vi "Stop.vi"(8 "error in (no error)":errorcluster, 11 "MicronManager in":refnum<class "MicronManager.lvclass">) -> (0 "error out":errorcluster, 3 "MicronManager out":refnum<class "MicronManager.lvclass">)   [LabVIEW 2019, in "MicronManager.lvclass"]
uses:
  MicronManager.lvclass
  MicronManager.lvclass/MicronManager.ctl
  <vilib>/SLL Toolkit/SLL Easy TCP/_SubVIs/TCP Initialize Client - Local.vi
  <vilib>/SLL Toolkit/SLL Easy TCP/SLL Easy API via TCP.lvclass
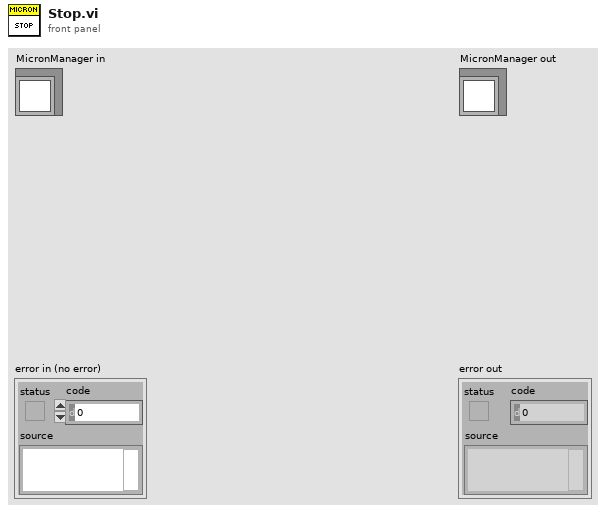
[diagram p1: front panel]
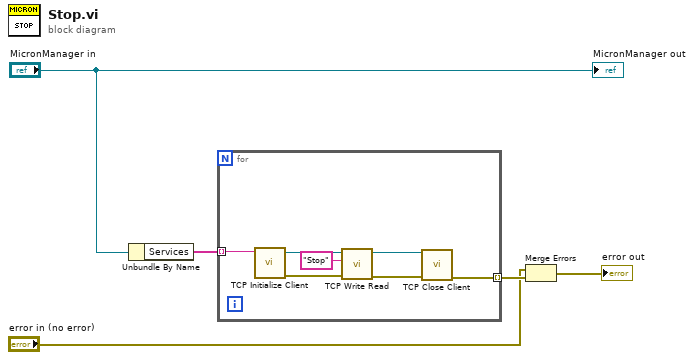
[diagram p0: block diagram]
diagram:
  n1 = Unbundle By Name("MicronManager in") -> ("Services"=w1:string[])
  n2 = for {
    tunnel: w1 -> [w7] mode=indexing
    tunnel: [w8] -> w4 mode=indexing
    n3 = call-poly <vilib>:"TCP Initialize Client.vi"("Service Name"=w7) -> ("error out"=w11:errorcluster, "connection ID Out"=w9:refnum<k5>)  [unwired: 9 in]
    n4 = call <vilib>:"TCP Write Read.vi"("error in (no error)"=w11, "Write Data"="Stop", "connection ID In"=w9) -> ("error out"=w12:errorcluster, "connection ID Out"=w10:refnum<k5>)  [unwired: 5 in, 2 out]
    n5 = call <vilib>:"TCP Close Client.vi"("error in (no error)"=w12, "connection ID"=w10) -> ("error out"=w8:errorcluster)  [unwired: 9 in]
  }
  n6 = Merge Errors("error in (no error)", w4) -> (→"error out":errorcluster)
  "MicronManager out" <- "MicronManager in"
